vi "write can fd.vi"(5 "switch bitrate? (F)":bool, 7 "extended id? (F)":bool, 8 "error in (no error)":errorcluster, 9 "data":u8[](array[numeric]) format="%x", 10 "id":u32 format="%x", 11 "channel":u16 format="%x") -> (0 "error out":errorcluster)   [LabVIEW 2024, in "atsj peakcan basic.lvlib"]
doc: "Writes a CAN FD message through an FD-capable PeakCAN <b>channel</b>."
uses:
  atsj peakcan basic.lvlib
  support/x64/PCANBasic.dll
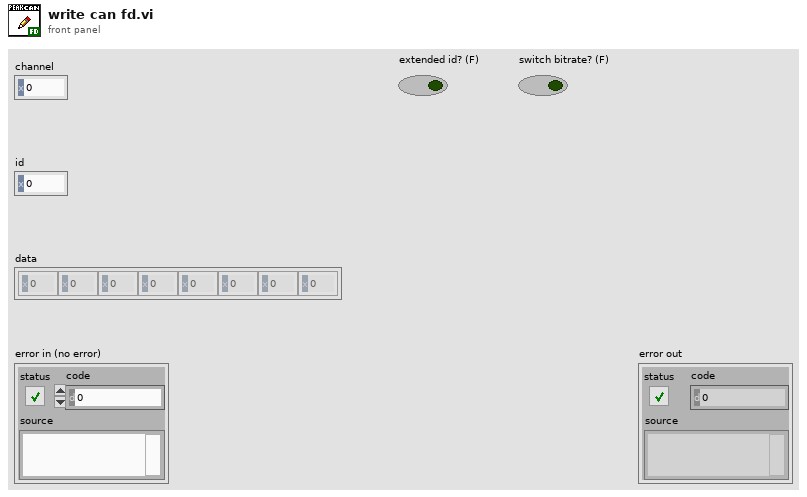
[diagram p1: front panel]
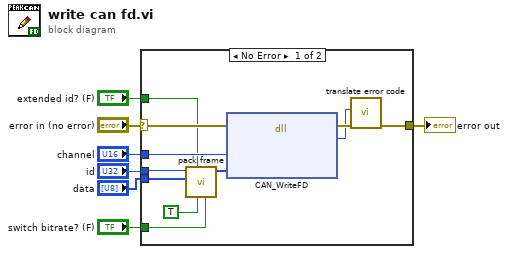
[diagram p0: block diagram]
diagram:
  n1 = case shown="No Error" "error in (no error)" {
    selector: "error in (no error)" -> [w14 w19]
    tunnel: "id" -> [w12 _]
    tunnel: "channel" -> [w18 _]
    tunnel: [w15 w19] -> w1
    tunnel: "data" -> [w11 _]
    tunnel: "extended id? (F)" -> [w10 _]
    tunnel: "switch bitrate? (F)" -> [w8 _]
    frame No Error {
      n2 = call "pack frame.vi"("switch bitrate? (F)"=w8, "can fd? (F)"=TRUE, "extended id?"=w10, "data"=w11, "id"=w12) -> ("frame"=w13:u8[])  [unwired: 6 in]
      n3 = dll-call lib="C:/atsj/plateau/atsj-peakcan-basic-for-labview/src/support/x64/PCANBasic.dll" fn="CAN_WriteFD" ("write can fd")(error in=w14, "Channel"=w18, "MessageBuffer"=w13) -> (error out=w17:errorcluster, "Status"=w16:u32)  [unwired: 4 in, 1 out]
      n4 = call "translate error code.vi"("error in (no error)"=w17, "error code"=w16) -> ("error out"=w15:errorcluster)  [unwired: 9 in]
    }
    frame Error {
    }
  }
  "error out" <- w1
